vi "XYtoStrings.vi"(10 "Array 2":dbl[](array[numeric]), 11 "Array":dbl[](array[numeric])) -> (3 "concatenated string":string)   [LabVIEW 2021]
panel:
  out "appended array":dbl[][](array[numeric])
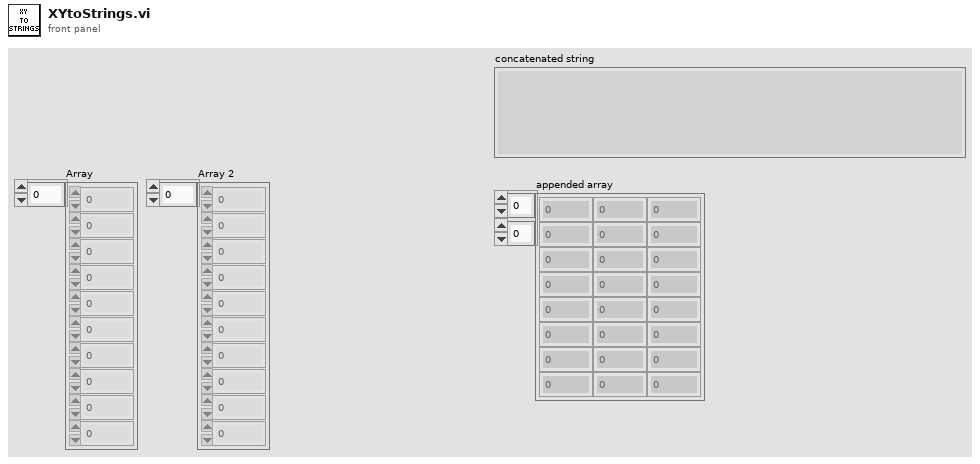
[diagram p1: front panel]
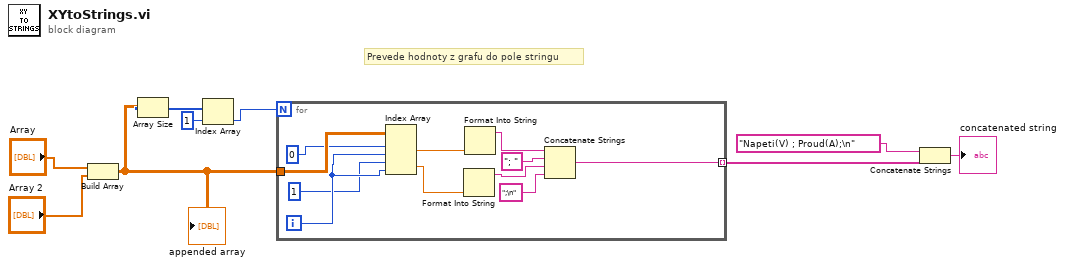
[diagram p0: block diagram]
diagram:
  # "Prevede hodnoty z grafu do pole stringu"
  n1 = Build Array("Array", "Array 2") -> (w4:dbl[][])
  "appended array" <- w4
  n2 = Array Size(array=w4) -> (size(s)=w7:i32[])
  n3 = Index Array(array=w7, index=1) -> (element=w5:i32)
  n4 = for {
    N: w5 -> [_]
    tunnel: w4 -> [w20]
    tunnel: [w13] -> w3 mode=indexing
    i -> [w11]
    n5 = Index Array(array=w20, index (row) #1=0 ("disabled index (col)"), index (col) #1=w11, index (row) #2=1 ("disabled index (col)"), index (col) #2=w11) -> (element #1=w19:dbl, element #2=w18:dbl)
    n6 = Format Into String(w18) -> (resulting string=w15:string)  [unwired: 3 in, 1 out]
    n7 = Format Into String(w19) -> (resulting string=w17:string)  [unwired: 3 in, 1 out]
    n8 = Concatenate Strings(w17, "; " ("string"), w15, ";\n" ("string")) -> (w13:string)
  }
  n9 = Concatenate Strings("Napeti(V) ; Proud(A);\n" ("string"), w3) -> (→"concatenated string":string)
